vi "PreBuildAction.vi"(6 "Top Level/Always Included VIs":path[](array[path]), 7 "Main Destination Path":path, 9 "Target Name":string, 10 "Build Specification Name":string, 11 "Project Path":path) -> (0 "error out":errorcluster)   [LabVIEW 2024]
uses:
  <vilib>/Utility/file.llb/Write Delimited Spreadsheet (string).vi
  <vilib>/AppBuilder/AB_API_Simple/NI_App_Builder_API.lvlib
  <vilib>/AppBuilder/AB_API_Simple/Get Build Specification Version (path).vi
  <vilib>/AppBuilder/AB_API_Simple/Set Build Specification Version (path).vi
  <vilib>/Utility/file.llb/Read Delimited Spreadsheet (string).vi
  Typdefinitionen & Beschreibung/PreBuildActionZustand.ctl
  Typdefinitionen & Beschreibung/PreBuildActionCluster.ctl
  <vilib>/AppBuilder/AB_API_Simple/Build Specification Version.ctl
panel:
  out "Version:":string
  in  "OK":bool
  in  "Vorgenommene Änderungen in dieser Build-Nr.":string
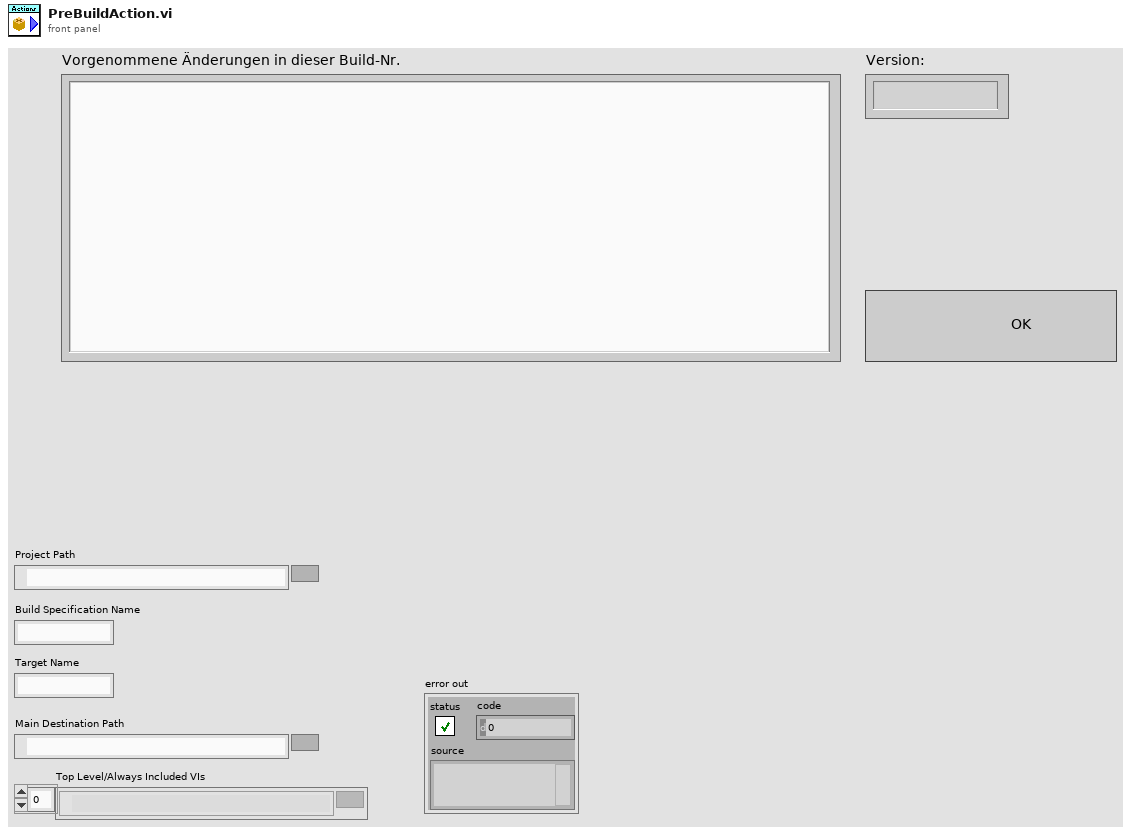
[diagram p1: front panel]
types:
  T1 = typedef "PreBuildActionCluster.ctl" = cluster{"Version aus Ordnername":string, "Major":u8, "Minor":u8, "Fix":u8, "Text für Version_Info.txt":string[], "Kommentar eingegeben?":bool}
  T2 = typedef "PreBuildActionZustand.ctl" = enum16{"Version in Ordnername auslesen & kontrollieren", "Prüfen ob Version schon einmal übersetzt wurde", "Neue Version setzen und Build abbrechen", "Auf Eingabe von User warten", "Version_Info.txt aktualisieren"}
  T3 = typedef "NI_App_Builder_API.lvlib/Build Specification Version.ctl" = cluster{"Major":u16, "Minor":u16, "Fix":u16, "Build":u16}
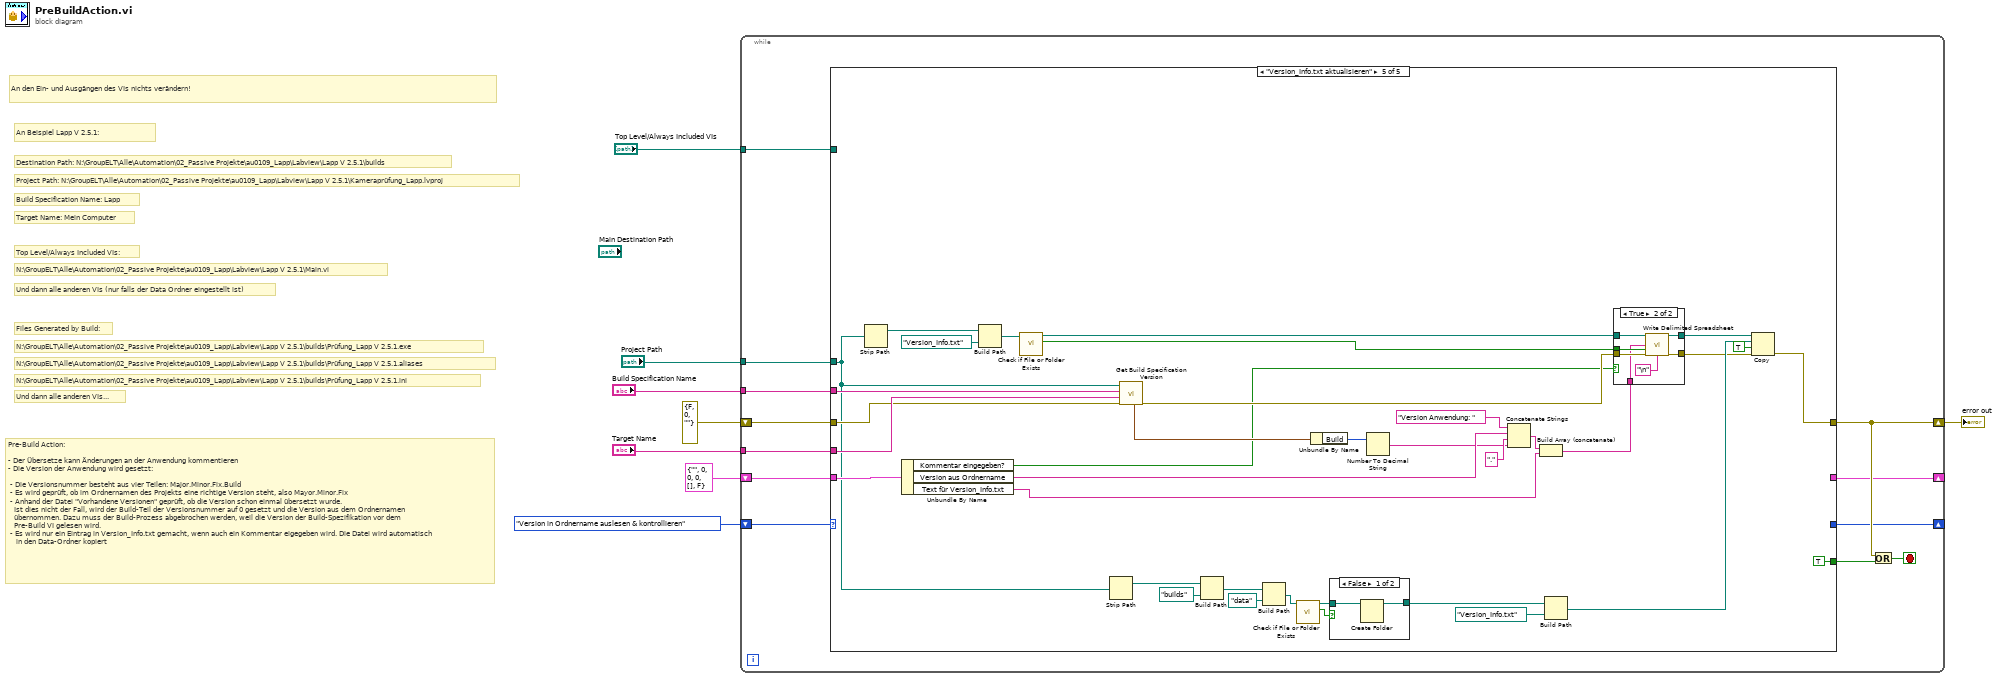
[diagram p0: block diagram]
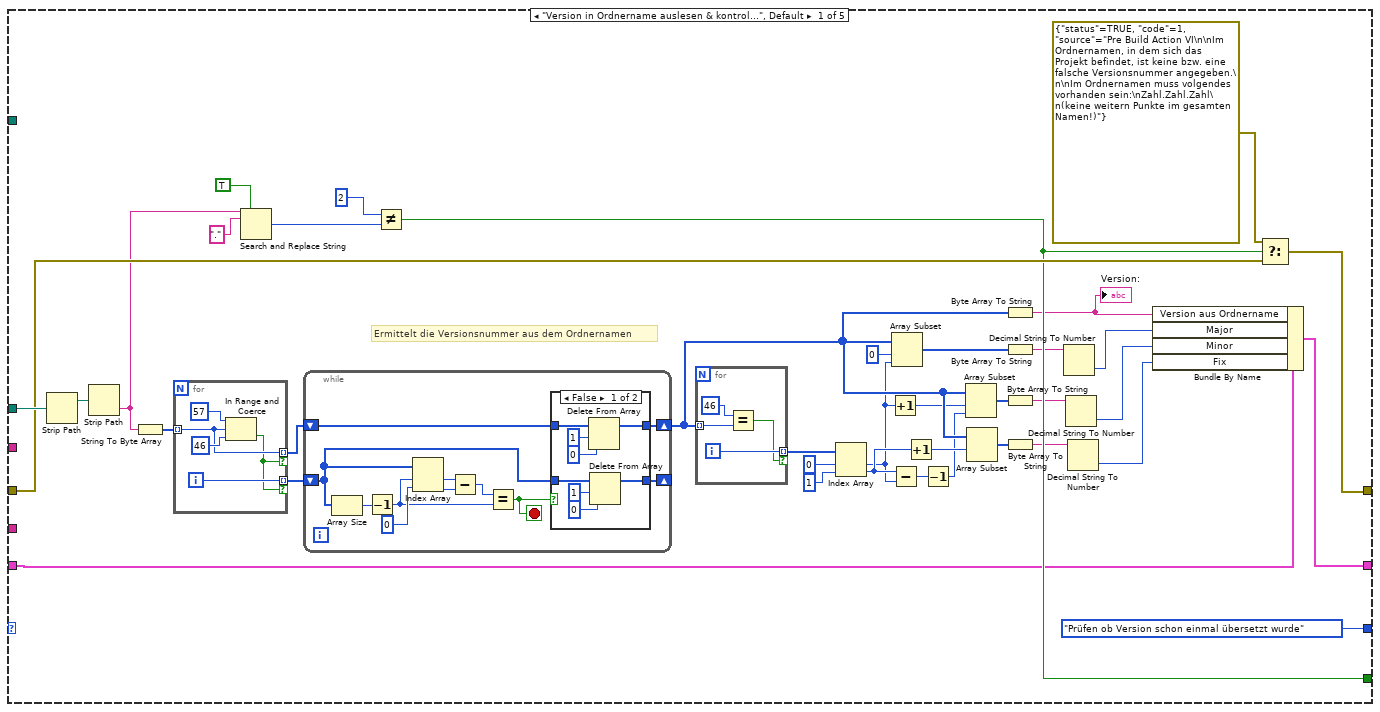
[diagram p2: hidden frame]
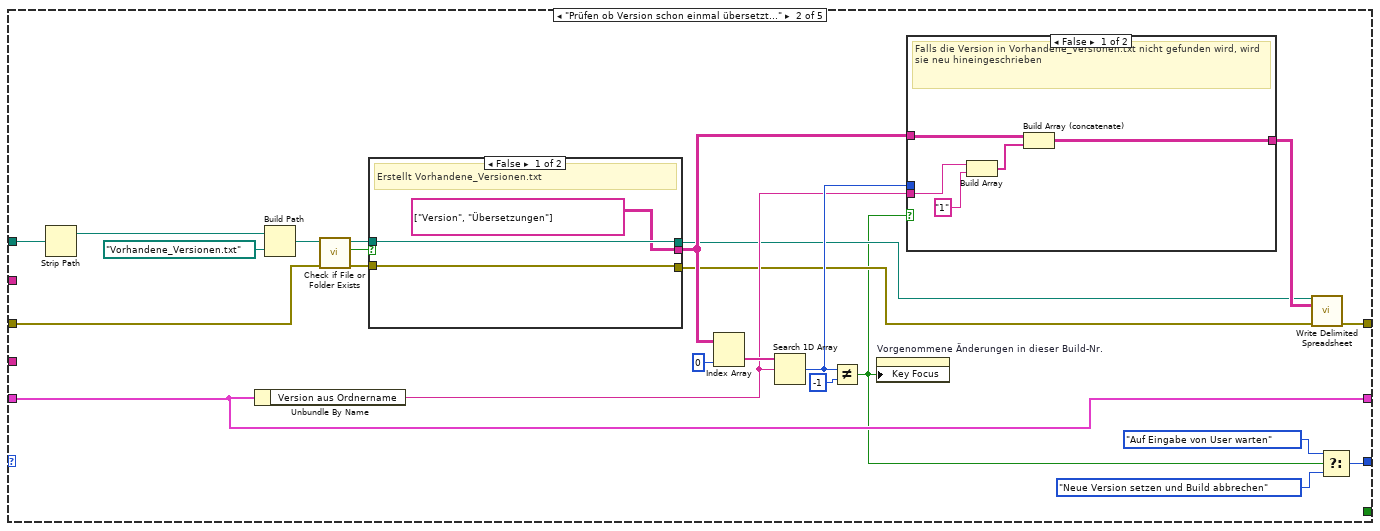
[diagram p4: hidden frame]
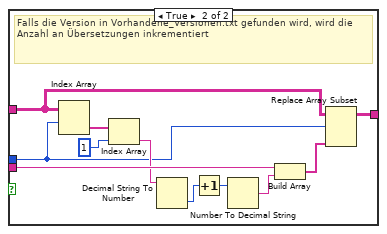
[diagram p5: hidden frame]
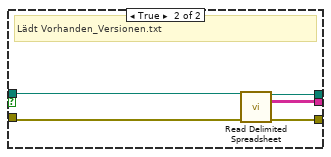
[diagram p6: hidden frame]
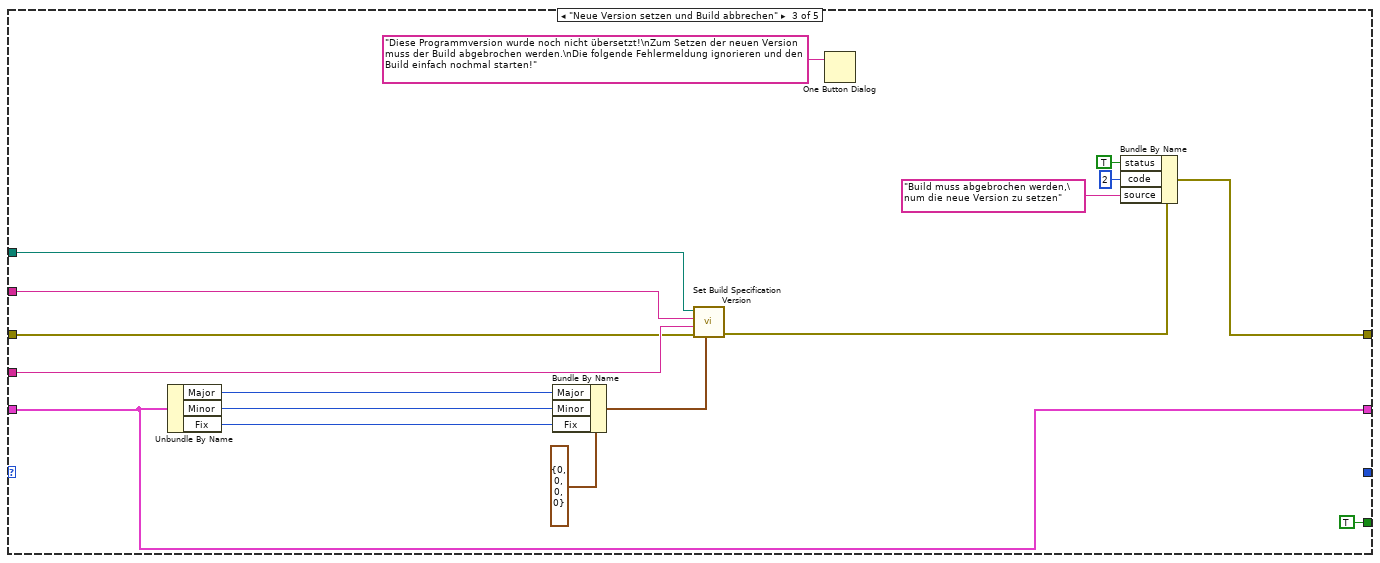
[diagram p7: hidden frame]
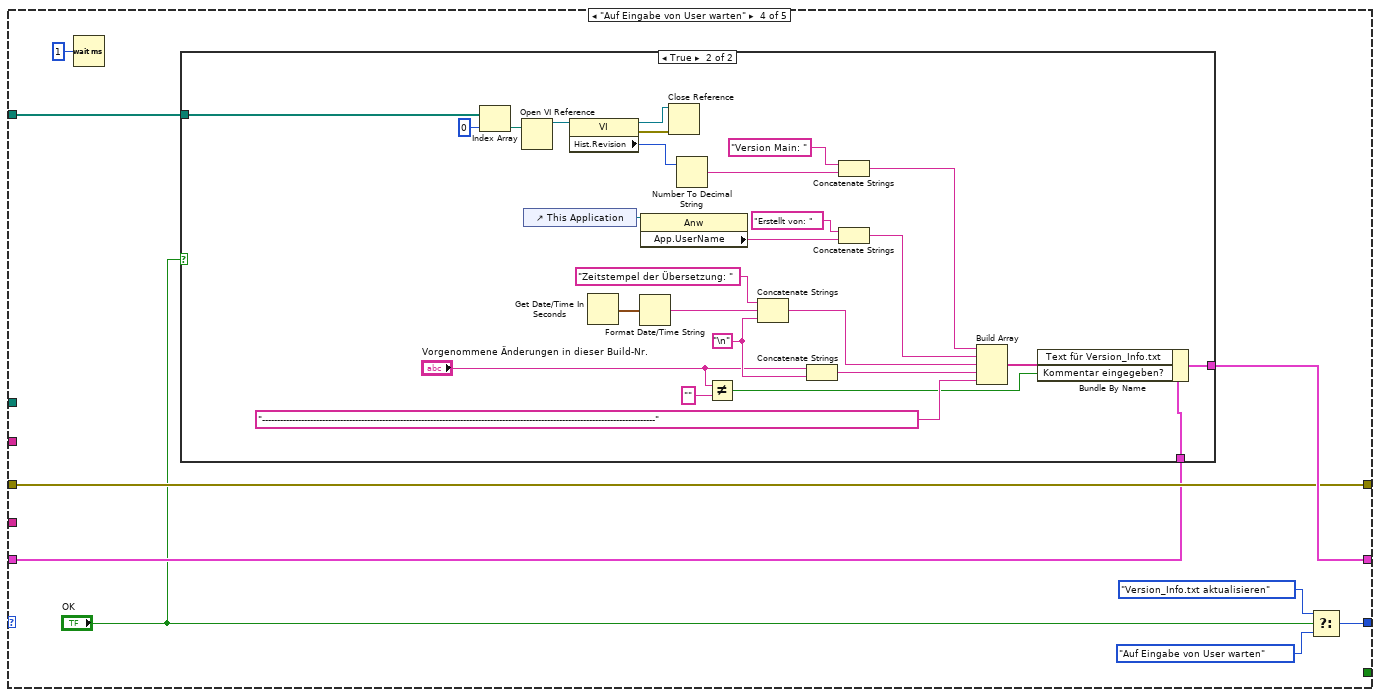
[diagram p8: hidden frame]
diagram:
  # "Pre-Build Action:\n\n- Der Übersetze kann Änderungen an der Anwendung kommentieren\n- Die Version der Anwendung wird gesetzt:\n\n\t- Die Versionsnummer besteht aus vier Teilen: Major.Minor.Fix.Build\n - Es wird geprüft, ob im Ordnernamen des Projekts eine richtige Version steht, also Mayor.Minor.Fix\n\t- Anhand der Datei \"Vorhandene Versionen\" geprüft, ob die Version schon einmal übersetzt wurde.\n\t  Ist dies nicht der Fall, wird der Build-Teil der Versionsnummer auf 0 gesetzt und die Version aus dem Ordnernamen\n   übernommen. Dazu muss der Build-Prozess abgebrochen werden, weil die Version der Build-Spezifikation vor dem \n   Pre-Build VI gelesen wird.\n - Es wird nur ein Eintrag in Version_Info.txt gemacht, wenn auch ein Kommentar eigegeben wird. Die Datei wird automatisch\n    in den Data-Ordner kopiert"
  # "An den Ein- und Ausgängen des VIs nichts verändern!"
  # "Files Generated by Build:"
  # "N:\\GroupELT\\Alle\\Automation\\02_Passive Projekte\\au0109_Lapp\\Labview\\Lapp V 2.5.1\\Main.vi"
  # "Top Level/Always Included VIs:"
  # "Target Name: Mein Computer"
  # "Build Specification Name: Lapp"
  # "Project Path: N:\\GroupELT\\Alle\\Automation\\02_Passive Projekte\\au0109_Lapp\\Labview\\Lapp V 2.5.1\\Kameraprüfung_Lapp.lvproj"
  # "Destination Path: N:\\GroupELT\\Alle\\Automation\\02_Passive Projekte\\au0109_Lapp\\Labview\\Lapp V 2.5.1\\builds"
  # "An Beispiel Lapp V 2.5.1:"
  # "Und dann alle anderen VIs (nur falls der Data Ordner eingestellt ist)"
  # "Und dann alle anderen VIs..."
  # "N:\\GroupELT\\Alle\\Automation\\02_Passive Projekte\\au0109_Lapp\\Labview\\Lapp V 2.5.1\\builds\\Prüfung_Lapp V 2.5.1.ini"
  # "N:\\GroupELT\\Alle\\Automation\\02_Passive Projekte\\au0109_Lapp\\Labview\\Lapp V 2.5.1\\builds\\Prüfung_Lapp V 2.5.1.aliases"
  # "N:\\GroupELT\\Alle\\Automation\\02_Passive Projekte\\au0109_Lapp\\Labview\\Lapp V 2.5.1\\builds\\Prüfung_Lapp V 2.5.1.exe"
  n1 = while {
    tunnel: "Project Path" -> [w18]
    shift-right: [w15] -> w1
    shift-left: errorcluster {"status"=FALSE, "code"=0, "source"=""} ("error constant") -> [w19]
    shift-right: [w14] -> _
    shift-left: PreBuildActionZustand."Version in Ordnername auslesen & kontrollieren" -> [w20]
    shift-right: [w12] -> _
    shift-left: T1 {"Version aus Ordnername"="", "Major"=0, "Minor"=0, "Fix"=0, "Text für Version_Info.txt"=[], "Kommentar eingegeben?"=FALSE} -> [w13]
    tunnel: "Target Name" -> [w11]
    tunnel: "Build Specification Name" -> [w10]
    tunnel: "Top Level/Always Included VIs" -> [w9]
    stop <- w17 stop-if-true
    n2 = case shown="\"Version_Info.txt aktualisieren\"" w20 {
      tunnel: w19 -> [w51 w105 w149 w157 w213]
      tunnel: w18 -> [w53 w107 w152 _ w206]
      tunnel: [w50 w95 w140 w157 w202] -> w15
      tunnel: [w49 _ TRUE _ TRUE] -> w16
      tunnel: [PreBuildActionZustand."Prüfen ob Version schon einmal übersetzt wurde" w91 _ w159 _] -> w14
      tunnel: w13 -> [w47 w93 w142 w155 w212]
      tunnel: [w46 w93 w142 w158 _] -> w12
      tunnel: w11 -> [_ _ w150 _ w215]
      tunnel: w10 -> [_ _ w151 _ w211]
      tunnel: w9 -> [_ _ _ w154 _]
      frame "Version in Ordnername auslesen & kontrollieren", Default {
        # "Ermittelt die Versionsnummer aus dem Ordnernamen"
        n3 = Strip Path(path=w53) -> (stripped path=w54:path)  [unwired: 1 out]
        n4 = Strip Path(path=w54) -> (name=w28:string)  [unwired: 1 out]
        n5 = String To Byte Array(string=w28) -> (unsigned byte array=w39:u8[])
        n6 = for {
          tunnel: w39 -> [w86] mode=indexing
          tunnel: [w86] -> w43 mode=indexing if=w84
          tunnel: [w85] -> w45 mode=indexing if=w84
          i -> [w85]
          n7 = In Range and Coerce(upper limit=u8 57, x=w86, lower limit=u8 46) -> (In Range?=w84:bool)  [unwired: 1 out]
        }
        n8 = Search and Replace String(replace all?=TRUE ("Alle ersetzen? (F)"), input string=w28, search string=".") -> (number of replacements=w56:i32)  [unwired: 5 in, 3 out]
        n9 = while {
          shift-right: [w65] -> w44
          shift-left: w43 -> [w66]
          shift-right: [w63] -> _
          shift-left: w45 -> [w64]
          stop <- w67 stop-if-true
          n10 = Array Size(array=w64) -> (size(s)=w62:i32)
          n11 = Decrement(x=w62) -> (x-1=w59:i32)
          n12 = Index Array(array=w64, index #1=w59, index #2=0 ("index")) -> (element #1=w69:i32, element #2=w68:i32)
          n13 = Subtract(x=w69, y=w68) -> (x-y=w61:i32)
          n14 = Equal?(x=w61, y=w59) -> (x = y?=w67:bool)
          n15 = case shown="False" w67 {
            tunnel: w66 -> [w77 w79]
            tunnel: [w74 w79] -> w65
            tunnel: w64 -> [w71 w78]
            tunnel: [w70 w78] -> w63
            frame False {
              n16 = Delete From Array(array=w77, length=1, index=0) -> (array with subset deleted=w74:u8[])  [unwired: 1 out]
              n17 = Delete From Array(array=w71, length=1, index=0) -> (array with subset deleted=w70:i32[])  [unwired: 1 out]
            }
            frame True {
            }
          }
        }
        n18 = Not Equal?(x=2, y=w56) -> (x != y?=w49:bool)
        n19 = for {
          tunnel: w44 -> [w83] mode=indexing
          tunnel: [w81] -> w32 mode=indexing if=w80
          i -> [w81]
          n20 = Equal?(x=u8 46, y=w83) -> (x = y?=w80:bool)
        }
        n21 = Index Array(array=w32, index #1=0 ("index"), index #2=1 ("index")) -> (element #1=w34:i32, element #2=w37:i32)
        n22 = Increment(x=w34) -> (x+1=w33:i32)
        n23 = Subtract(x=w37, y=w34) -> (x-y=w35:i32)
        n24 = Array Subset(array=w44, index=0, length=w34) -> (w40:u8[])
        n25 = Increment(x=w37) -> (x+1=w38:i32)
        n26 = Decrement(x=w35) -> (x-1=w36:i32)
        n27 = Array Subset(array=w44, index=w33, length=w36) -> (w41:u8[])
        n28 = Array Subset(array=w44, index=w38) -> (w42:u8[])  [unwired: 1 in]
        n29 = Byte Array To String(unsigned byte array=w44) -> (string=w21:string)
        "Version:" <- w21
        n30 = Byte Array To String(unsigned byte array=w40) -> (string=w27:string)
        n31 = Byte Array To String(unsigned byte array=w41) -> (string=w26:string)
        n32 = Byte Array To String(unsigned byte array=w42) -> (string=w25:string)
        n33 = Decimal String To Number(string=w27) -> (number=w24:i32)  [unwired: 2 in, 1 out]
        n34 = Decimal String To Number(string=w26) -> (number=w23:i32)  [unwired: 2 in, 1 out]
        n35 = Decimal String To Number(string=w25) -> (number=w22:i32)  [unwired: 2 in, 1 out]
        n36 = Bundle By Name(cluster=w47, "Version aus Ordnername"=w21, "Major"=w24, "Minor"=w23, "Fix"=w22) -> (w46:T1)
        n37 = Select(t=errorcluster {"status"=TRUE, "code"=1, "source"="Pre Build Action VI\n\nIm Ordnernamen, in dem sich das Projekt befindet, ist keine bzw. eine falsche Versionsnummer angegeben.\n\nIm Ordnernamen muss volgendes vorhanden sein:\nZahl.Zahl.Zahl\n(keine weitern Punkte im gesamten Namen!)"} ("error constant"), s=w49, f=w51) -> (s? t:f=w50:errorcluster)
      }
      frame "Prüfen ob Version schon einmal übersetzt wurde" {
        n38 = Strip Path(path=w107) -> (stripped path=w106:path)  [unwired: 1 out]
        n39 = Unbundle By Name(w93) -> ("Version aus Ordnername"=w98:string)
        n40 = Build Path(base path=w106, name or relative path=path "Vorhandene_Versionen.txt" ("Name oder relativer Pfad")) -> (appended path=w108:path)
        n41 = call <vilib>:"Check if File or Folder Exists.vi"("error in (no error)"=w105, "path"=w108) -> ("error out"=w104:errorcluster, "file or folder exists?"=w110:bool, "dup path"=w109:path)  [unwired: 7 in]
        n42 = case shown="False" w110 {
          tunnel: [string[][] [["Version", "Übersetzungen"]] ("all rows") w135] -> w100
          tunnel: w109 -> [w130 w134]
          tunnel: [w130 w133] -> w94
          tunnel: [w128 w132] -> w96
          tunnel: w104 -> [w128 w131]
          frame False {
            # "Erstellt Vorhandene_Versionen.txt"
          }
          frame True {
            # "Lädt Vorhanden_Versionen.txt"
            n43 = call-poly <vilib>:"Read Delimited Spreadsheet.vi"("file path (dialog if empty)"=w134, "error in (no error)"=w131) -> ("new file path (Not A Path if cancelled)"=w133:path, "all rows"=w135:string[][], "error out"=w132:errorcluster)  [unwired: 8 in, 3 out]
          }
        }
        n44 = Index Array(array=w100, index (col)=0 ("disabled index (col)")) -> (element=w101:string[])  [unwired: 1 in]
        n45 = Search 1D Array(1D array=w101, element=w98) -> (index of element=w99:i32)  [unwired: 1 in]
        n46 = Not Equal?(x=w99, y=-1) -> (x != y?=w89:bool)
        n47 = property on="Vorgenommene Änderungen in dieser Build-Nr." class="Str"("Key Focus"=w89) -> ()  [unwired: 2 in, 2 out]
        n48 = case shown="False" w89 {
          tunnel: w100 -> [w115 w118]
          tunnel: [w116 w124] -> w97
          tunnel: w98 -> [w114 w125]
          tunnel: w99 -> [_ w117]
          frame False {
            # "Falls die Version in Vorhandene_Versionen.txt nicht gefunden wird, wird sie neu hineingeschrieben"
            n49 = Build Array(w114, "1" ("element")) -> (w112:string[])
            n50 = Build Array (concatenate)(w115, w112) -> (w116:string[][])
          }
          frame True {
            # "Falls die Version in Vorhandene_Versionen.txt gefunden wird, wird die Anzahl an Übersetzungen inkrementiert"
            n51 = Index Array(array=w118, index (row)=w117) -> (element=w121:string[])  [unwired: 1 in]
            n52 = Index Array(array=w121, index=1) -> (element=w119:string)
            n53 = Decimal String To Number(string=w119) -> (number=w127:i32)  [unwired: 2 in, 1 out]
            n54 = Increment(x=w127) -> (x+1=w126:i32)
            n55 = Number To Decimal String(number=w126) -> (decimal integer string=w123:string)  [unwired: 1 in]
            n56 = Build Array(w125, w123) -> (w122:string[])
            n57 = Replace Array Subset(array=w118, new element=w122, index (row)=w117) -> (w124:string[][])  [unwired: 1 in]
          }
        }
        n58 = call-poly <vilib>:"Write Delimited Spreadsheet.vi"("file path (dialog if empty)"=w94, "2D data"=w97, "error in (no error)"=w96) -> ("error out"=w95:errorcluster)  [unwired: 11 in, 1 out]
        n59 = Select(t=PreBuildActionZustand."Auf Eingabe von User warten", s=w89, f=PreBuildActionZustand."Neue Version setzen und Build abbrechen") -> (s? t:f=w91:T2)
      }
      frame "Neue Version setzen und Build abbrechen" {
        n60 = Unbundle By Name(w142) -> ("Major"=w147:u8, "Minor"=w146:u8, "Fix"=w145:u8)
        n61 = Bundle By Name(cluster=T3 {"Major"=0, "Minor"=0, "Fix"=0, "Build"=0} ("Build Specification Version"), "Major"=w147, "Minor"=w146, "Fix"=w145) -> (w144:T3)
        n62 = call-poly <vilib>:"Set Build Specification Version.vi"("Build Specification Version"=w144, "error in (no error)"=w149, "Name of target (My Computer)"=w150, "Name of build specification"=w151, "Path to project"=w152) -> ("error out"=w141:errorcluster)  [unwired: 6 in]
        n63 = One Button Dialog(message="Diese Programmversion wurde noch nicht übersetzt!\nZum Setzen der neuen Version muss der Build abgebrochen werden.\nDie folgende Fehlermeldung ignorieren und den Build einfach nochmal starten!") -> ()  [unwired: 1 in, 1 out]
        n64 = Bundle By Name(cluster=w141, "status"=TRUE, "code"=2, "source"="Build muss abgebrochen werden,\num die neue Version zu setzen") -> (w140:errorcluster)
      }
      frame "Auf Eingabe von User warten" {
        n65 = Wait (ms)(milliseconds to wait=u32 1 ("Zu wartende ms")) -> ()  [unwired: 1 out]
        n66 = case shown="True" "OK" {
          tunnel: [w162 w189] -> w158
          tunnel: w155 -> [w162 w184]
          tunnel: w154 -> [_ w174]
          frame False {
          }
          frame True {
            w166 = "\n"
            n67 = Index Array(array=w174, index=0) -> (element=w178:path)
            n68 = Open VI Reference(vi path=w178) -> (vi reference=w183:refnum<vi>)  [unwired: 5 in, 1 out]
            n69 = control-ref of="This Application"() -> (w188:refnum<vi>)
            n70 = property class="VI"(reference=w183) -> (reference out=w180:refnum<vi>, error out=w181:errorcluster, "Hist.Revision"=w182:u32)  [unwired: 1 in]
            n71 = Get Date/Time In Seconds() -> (seconds since 1Jan1904=w173:timestamp)
            n72 = Format Date/Time String(seconds (now)=w173) -> (date/time string=w172:string)  [unwired: 2 in]
            n73 = property class="Anw"(reference=w188) -> ("App.UserName"=w187:string)  [unwired: 1 in, 2 out]
            n74 = Close Reference(reference=w180, error in (no error)=w181) -> ()  [unwired: 1 out]
            n75 = Number To Decimal String(number=w182) -> (decimal integer string=w179:string)  [unwired: 1 in]
            n76 = Not Equal?(x="Vorgenommene Änderungen in dieser Build-Nr.", y="") -> (x != y?=w163:bool)
            n77 = Concatenate Strings("Zeitstempel der Übersetzung: " ("String"), w172, w166) -> (w170:string)
            n78 = Concatenate Strings("Vorgenommene Änderungen in dieser Build-Nr.", w166) -> (w167:string)
            n79 = Concatenate Strings("Version Main: " ("String"), w179) -> (w175:string)
            n80 = Concatenate Strings("Erstellt von: " ("String"), w187) -> (w169:string)
            n81 = Build Array(w175, w169, w170, w167, "-----------------------------------------------------------------------------------------------------------------------------------" ("Element")) -> (w185:string[])
            n82 = Bundle By Name(cluster=w184, "Text für Version_Info.txt"=w185, "Kommentar eingegeben?"=w163) -> (w189:T1)
          }
        }
        n83 = Select(t=PreBuildActionZustand."Version_Info.txt aktualisieren", s="OK", f=PreBuildActionZustand."Auf Eingabe von User warten") -> (s? t:f=w159:T2)
      }
      frame "Version_Info.txt aktualisieren" {
        n84 = Strip Path(path=w206) -> (stripped path=w205:path)  [unwired: 1 out]
        n85 = Unbundle By Name(w212) -> ("Kommentar eingegeben?"=w190:bool, "Version aus Ordnername"=w210:string, "Text für Version_Info.txt"=w209:string[])
        n86 = Build Path(base path=w205, name or relative path=path "Version_Info.txt" ("Name oder relativer Pfad")) -> (appended path=w207:path)
        n87 = call <vilib>:"Check if File or Folder Exists.vi"("path"=w207) -> ("file or folder exists?"=w204:bool, "dup path"=w203:path)  [unwired: 8 in, 1 out]
        n88 = Strip Path(path=w206) -> (stripped path=w214:path)  [unwired: 1 out]
        n89 = call-poly <vilib>:"Get Build Specification Version.vi"("error in (no error)"=w213, "Name of target (My Computer)"=w215, "Name of build specification"=w211, "Path to project"=w206) -> ("error out"=w201:errorcluster, "Build Specification Version"=w194:T3)  [unwired: 6 in]
        n90 = Build Path(base path=w214, name or relative path=path "builds") -> (appended path=w222:path)
        n91 = Build Path(base path=w222, name or relative path=path "data" ("Name oder relativer Pfad")) -> (appended path=w220:path)
        n92 = call <vilib>:"Check if File or Folder Exists.vi"("path"=w220) -> ("file or folder exists?"=w219:bool, "dup path"=w218:path)  [unwired: 8 in, 1 out]
        n93 = Unbundle By Name(w194) -> ("Build"=w200:u16)
        n94 = case shown="False" w219 {
          tunnel: w218 -> [w236 w237]
          tunnel: [w235 w237] -> w217
          frame False {
            n95 = Create Folder(path (use dialog)=w236) -> (created path=w235:path)  [unwired: 2 in, 2 out]
          }
          frame True {
          }
        }
        n96 = Number To Decimal String(number=w200) -> (decimal integer string=w195:string)  [unwired: 1 in]
        n97 = Concatenate Strings("Version Anwendung: " ("string"), w210, "." ("string"), w195) -> (w198:string)
        n98 = Build Array (concatenate)(w198, w209) -> (w197:string[])
        n99 = Build Path(base path=w217, name or relative path=path "Version_Info.txt" ("Name oder relativer Pfad")) -> (appended path=w216:path)
        n100 = case shown="True" w190 {
          tunnel: w204 -> [_ w234]
          tunnel: w203 -> [w227 w233]
          tunnel: w201 -> [w226 w232]
          tunnel: w197 -> [_ w231]
          tunnel: [w227 w230] -> w193
          tunnel: [w226 w229] -> w191
          frame False {
          }
          frame True {
            n101 = call-poly <vilib>:"Write Delimited Spreadsheet.vi"("file path (dialog if empty)"=w233, "1D data"=w231, "append to file? (new file:F)"=w234, "error in (no error)"=w232, "delimiter (\\t)"="\n") -> ("new file path (Not A Path if cancelled)"=w230:path, "error out"=w229:errorcluster)  [unwired: 9 in]
          }
        }
        n102 = Copy(8:w191, 9:TRUE ("Überschreiben (F)"), 10:w216, 11:w193) -> (0:w202:errorcluster)  [unwired: 1 in, 2 out]
      }
    }
    n103 = Or(x=w15, y=w16) -> (x .or. y?=w17:bool)
  }
  "error out" <- w1
